vi "appendXMLCorrectionParameters.vi"(8 "Correction Parameters":cluster{"X":sgl, "Y":sgl, "Movement Type":u16}, 9 "error in (no error)":errorcluster, 10 "Parent Camera Node":refnum<k20>, 11 "DOM document in":refnum<k20>) -> (0 "error out":errorcluster)   [LabVIEW 2013]
uses:
  <resource>/objmgr/DOMUserDefRef.rc
panel:
  out "Movement Type":u16
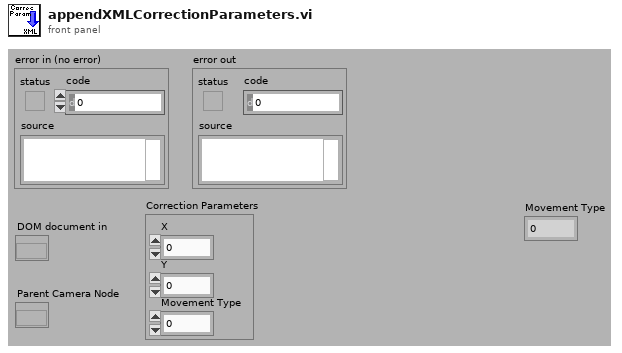
[diagram p1: front panel]
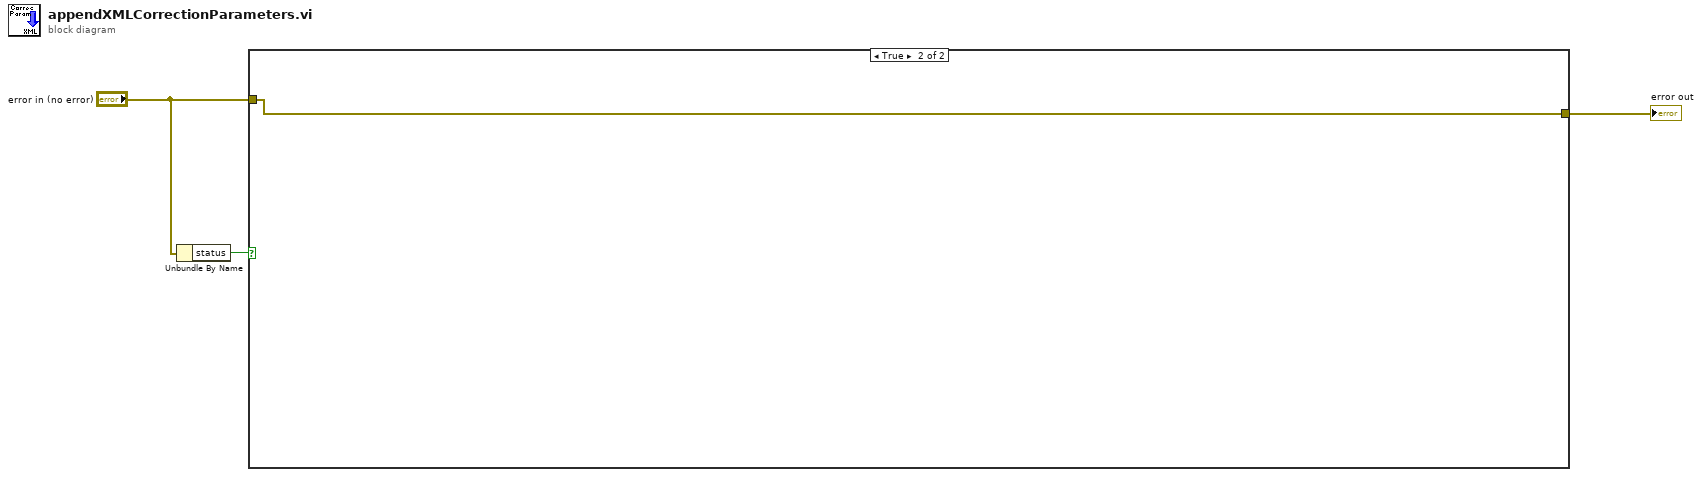
[diagram p0: block diagram]
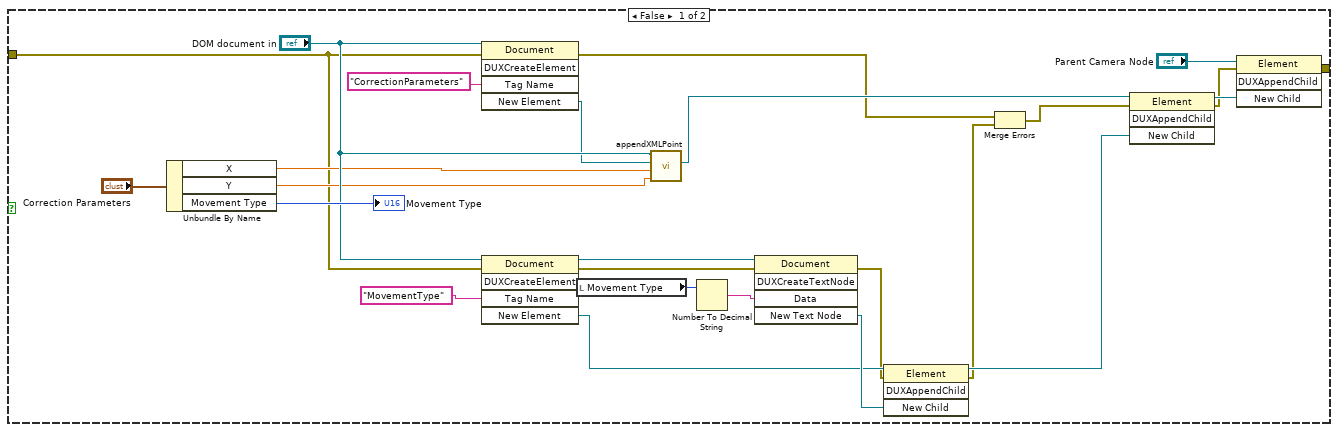
[diagram p2: hidden frame]
diagram:
  n1 = Unbundle By Name("error in (no error)") -> ("status"=w2:bool)
  n2 = case shown="True" w2 {
    tunnel: "error in (no error)" -> [w11 w29]
    tunnel: [w4 w29] -> w3
    frame False {
      n3 = Unbundle By Name("Correction Parameters") -> ("X"=w15:sgl, "Y"=w14:sgl, "Movement Type"=→"Movement Type":u16)
      n4 = invoke class="Document" method="DUXCreateElement"(reference="DOM document in", error in=w11, "Tag Name"="CorrectionParameters") -> (error out=w8:errorcluster, "New Element"=w13:refnum<k20>)  [unwired: 2 in, 3 out]
      n5 = invoke class="Document" method="DUXCreateElement"(reference="DOM document in", error in=w11, "Tag Name"="MovementType") -> (reference out=w26:refnum<k20>, error out=w10:errorcluster, "New Element"=w24:refnum<k20>)  [unwired: 2 in, 2 out]
      n6 = local read "Movement Type"() -> (w21:u16)
      n7 = call "appendXMLPoint.vi"("y"=w14, "x"=w15, "Parent Node"=w13, "DOM document in"="DOM document in") -> ("Parent Node Out"=w12:refnum<k20>)  [unwired: 5 in, 1 out]
      n8 = Number To Decimal String(number=w21) -> (decimal integer string=w20:string)  [unwired: 1 in]
      n9 = invoke class="Document" method="DUXCreateTextNode"(reference=w26, error in=w10, "Data"=w20) -> (error out=w9:errorcluster, "New Text Node"=w25:refnum<k20>)  [unwired: 2 in, 3 out]
      n10 = invoke class="Element" method="DUXAppendChild"(reference=w24, error in=w9, "New Child"=w25) -> (reference out=w23:refnum<k20>, error out=w7:errorcluster)  [unwired: 1 in, 2 out]
      n11 = Merge Errors(w8, w7) -> (w6:errorcluster)
      n12 = invoke class="Element" method="DUXAppendChild"(reference=w12, error in=w6, "New Child"=w23) -> (reference out=w17:refnum<k20>, error out=w5:errorcluster)  [unwired: 1 in, 2 out]
      n13 = invoke class="Element" method="DUXAppendChild"(reference="Parent Camera Node", error in=w5, "New Child"=w17) -> (error out=w4:errorcluster)  [unwired: 1 in, 3 out]
    }
    frame True {
    }
  }
  "error out" <- w3
